vi "WIFI下载.vi"(9 "远程端口":u16, 10 "地址":string, 11 "程序":string[](array[string])) -> ()   [LabVIEW 2018]
uses:
  user32.dll
panel:
  out "进度":string
  out "下载中……":i32(slide)=-1 scale=-1.0..35.0
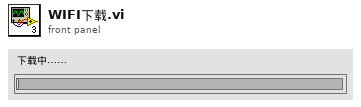
[diagram p1: front panel]
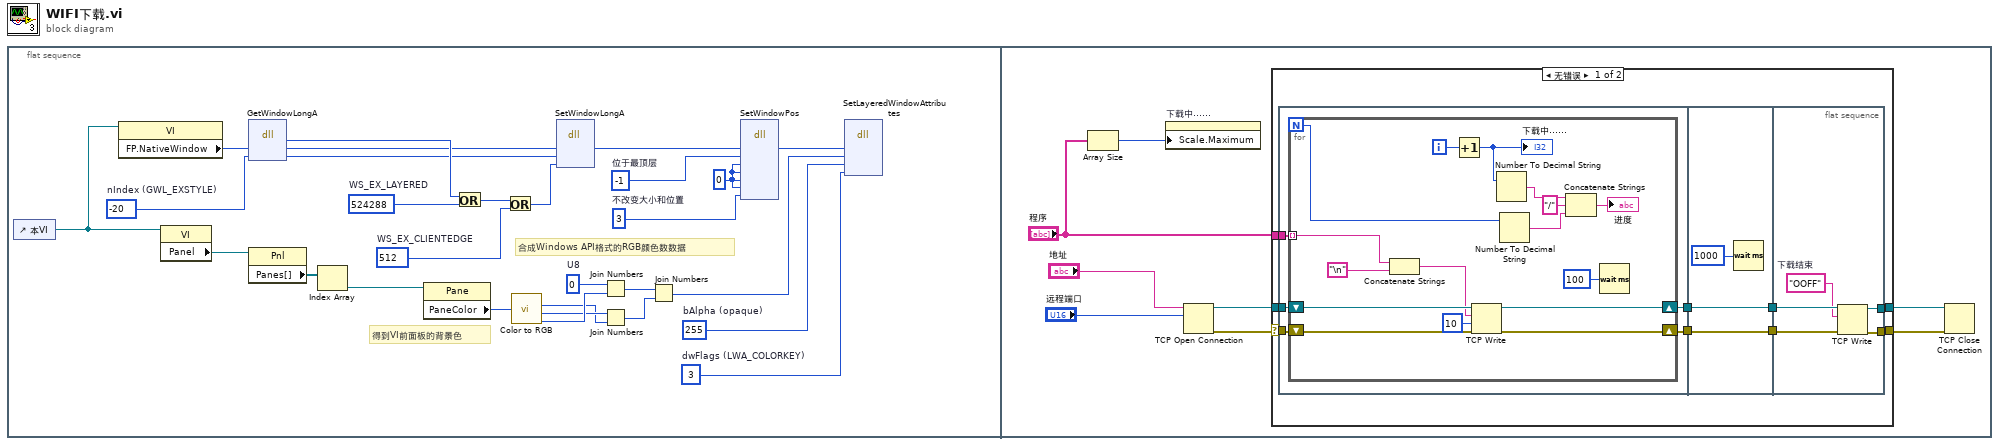
[diagram p0: block diagram]
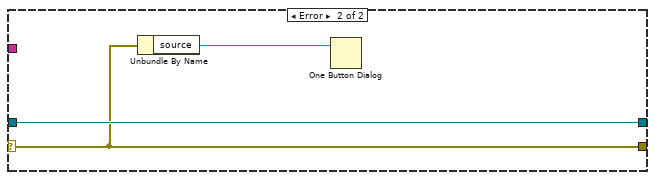
[diagram p2: hidden frame]
diagram:
  n1 = flat-sequence {
    frame #0 {
      w25 = 512  # WS_EX_CLIENTEDGE
      w21 = 3  # 不改变大小和位置
      w24 = 0 ("nIndex")
      w20 = -1  # 位于最顶层
      w2 = 255  # bAlpha (opaque)
      w1 = 3  # dwFlags (LWA_COLORKEY)
      w9 = u8 0  # U8
      w17 = 524288  # WS_EX_LAYERED
      w18 = -20  # nIndex (GWL_EXSTYLE)
      # "合成Windows API格式的RGB颜色数数据"
      # "得到VI前面板的背景色"
      n2 = control-ref of="本VI"() -> (w28:refnum<vi>)
      n3 = property class="VI"(reference=w28) -> ("FP.NativeWindow"=w19:u64)  [unwired: 1 in, 2 out]
      n4 = property class="VI"(reference=w28) -> ("Panel"=w4:refnum<vi>)  [unwired: 1 in, 2 out]
      n5 = dll-call lib="user32.dll" fn="GetWindowLongA"("handle"=w19, "nIndex"=w18) -> ("返回类型"=w16:i32, "handle"=w15:i32, "nIndex"=w14:i32)  [unwired: 3 in, 2 out]
      n6 = property class="Pnl"(reference=w4) -> ("Panes[]"=w5:refnum<vi>[])  [unwired: 1 in, 2 out]
      n7 = Index Array(array=w5) -> (element=w6:refnum<vi>)  [unwired: 1 in]
      n8 = property class="Pane"(reference=w6) -> ("PaneColor"=w10:u32)  [unwired: 1 in, 2 out]
      n9 = Or(x=w16, y=w17) -> (x .or. y?=w26:i32)
      n10 = Or(x=w26, y=w25) -> (x .or. y?=w27:i32)
      n11 = call <vilib>:"Color to RGB.vi"("Color"=w10) -> ("R"=w11:u8, "G"=w12:u8, "B"=w13:u8)  [unwired: 1 out]
      n12 = dll-call lib="USER32.DLL" fn="SetWindowLongA" label="SetWindowLong"("handle"=w15, "nIndex"=w14, "dwNewLong"=w27) -> ("handle"=w22:i32)  [unwired: 5 in, 3 out]
      n13 = Join Numbers(hi=w9, lo=w13) -> ((hi.lo)=w8:u16)
      n14 = Join Numbers(hi=w12, lo=w11) -> ((hi.lo)=w7:u16)
      n15 = Join Numbers(hi=w8, lo=w7) -> ((hi.lo)=w3:u32)
      n16 = dll-call lib="USER32.DLL" fn="SetWindowPos"("hWnd"=w22, "hWndInsertAfter"=w20, "x"=w24, "y"=w24, "cx"=w24, "cy"=w24, "wFlags"=w21) -> ("hWnd"=w23:i32)  [unwired: 9 in, 3 out]
      n17 = dll-call lib="USER32.DLL" fn="SetLayeredWindowAttributes" label="SetLayerdWindowAttributs"("handle"=w23, "crkey"=w3, "bAlpha"=w2, "dwFlags"=w1) -> ()  [unwired: 7 in, 3 out]
    }
    frame #1 {
      n18 = Array Size(array="程序") -> (size(s)=w30:i32)
      n19 = property on="下载中……" class="Slide (严格)"("Scale.Maximum"=w30) -> ()  [unwired: 2 in, 2 out]
      n20 = TCP Open Connection(address="地址", remote port or service name="远程端口") -> (connection ID=w36:refnum<k5>, error out=w31:errorcluster)  [unwired: 3 in]
      n21 = case shown="无错误" w31 {
        selector: w31 -> [w43 w76]
        tunnel: w36 -> [w45 w77]
        tunnel: [w37 w77] -> w35
        tunnel: [w38 w76] -> w34
        tunnel: "程序" -> [w44 _]
        frame No Error {
          n22 = flat-sequence {
            tunnel: w45 -> [w50]
            tunnel: w44 -> [w49]
            tunnel: w43 -> [w48]
            tunnel: [w47] -> w42
            tunnel: [w46] -> w41
            tunnel: w42 -> [w69]
            tunnel: w41 -> [w68]
            tunnel: [w69] -> w40
            tunnel: [w68] -> w39
            tunnel: w40 -> [w73]
            tunnel: w39 -> [w74]
            tunnel: [w72] -> w38
            tunnel: [w71] -> w37
            frame #0 {
              n23 = for {
                N -> [w52]
                shift-right: [w64] -> w47
                shift-left: w50 -> [w66]
                shift-right: [w63] -> w46
                shift-left: w48 -> [w65]
                tunnel: w49 -> [w62] mode=indexing
                i -> [w53]
                n24 = Concatenate Strings(w62, "\n") -> (w60:string)
                n25 = Increment(x=w53) -> (x+1=w58:i32)
                "下载中……" <- w58
                n26 = TCP Write(connection ID=w66, data in=w60, error in (no error)=w65, 9:10 ("超时毫秒(25000)")) -> (connection ID out=w64:refnum<k5>, error out=w63:errorcluster)  [unwired: 1 out]
                n27 = Number To Decimal String(number=w58) -> (decimal integer string=w57:string)  [unwired: 1 in]
                n28 = Number To Decimal String(number=w52) -> (decimal integer string=w55:string)  [unwired: 1 in]
                n29 = Concatenate Strings(w57, "/" ("字符串"), w55) -> (→"进度":string)
                n30 = Wait (ms)(milliseconds to wait=u32 100 ("等待时间（毫秒）")) -> ()  [unwired: 1 out]
              }
            }
            frame #1 {
              n31 = Wait (ms)(milliseconds to wait=u32 1000 ("等待时间（毫秒）")) -> ()  [unwired: 1 out]
            }
            frame #2 {
              w70 = "OOFF"  # 下载结束
              n32 = TCP Write(connection ID=w73, data in=w70, error in (no error)=w74) -> (connection ID out=w71:refnum<k5>, error out=w72:errorcluster)  [unwired: 1 in, 1 out]
            }
          }
        }
        frame Error {
          n33 = Unbundle By Name(w76) -> ("source"=w75:string)
          n34 = One Button Dialog(message=w75) -> ()  [unwired: 1 in, 1 out]
        }
      }
      n35 = TCP Close Connection(connection ID=w35, error in (no error)=w34) -> ()  [unwired: 1 in, 2 out]
    }
  }
